vi "Update Unicode Controls.vi"(8 "error in":errorcluster, 11 "String Refs":refnum<vi>[](array[refnum])) -> (0 "error out":errorcluster, 2 "Stop Event":refnum<user-event>, 3 "Value Change Event":refnum<user-event>)   [LabVIEW 2020, in "G-Unicode.lvlib"]
doc: "Launches a background task to monitor and update string controls in <b>String Refs</b> with the correct unicode value when a user types text. The caller MUST generate a user event using <b>Stop Event</b> to terminate the background task.\n\nDynamically register for <b>Value Change Event</b> to receive an event from any of the controls in <b>String Refs</b> after the unicode text has been applied. Use Read Control.vim with the ref from Value Change Event data to read the unicode text.\n\nAll controls in <b>String Refs</b> will have their Update While Typing? and Force Unicode Text properties set True."
uses:
  G-Unicode.lvlib
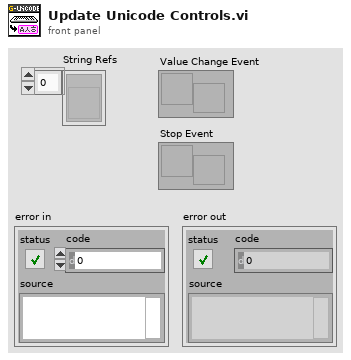
[diagram p1: front panel]
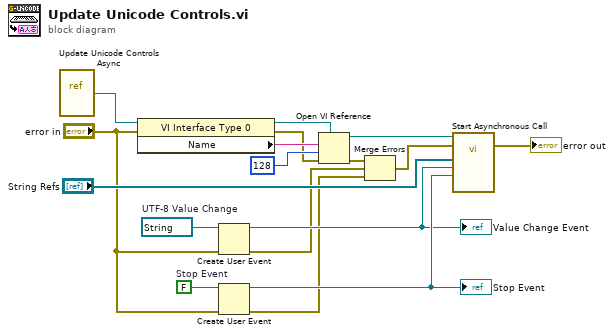
[diagram p0: block diagram]
diagram:
  w9 = refnum<vi> refnum  # UTF-8 Value Change
  w11 = FALSE  # Stop Event
  n1 = vi-ref "Update Unicode Controls Async.vi"() -> (w17:refnum<vi>)
  n2 = property class="VI Interface Type 0"(reference=w17, error in="error in") -> (reference out=w16:refnum<vi>, error out=w3:errorcluster, "Name"=w15:string)
  n3 = Create User Event(user event datatype=w9, error in="error in") -> (user event=w8:refnum<user-event>, error out=w5:errorcluster)
  "Value Change Event" <- w8
  n4 = Create User Event(user event datatype=w11, error in="error in") -> (user event=w10:refnum<user-event>, error out=w4:errorcluster)
  "Stop Event" <- w10
  n5 = Open VI Reference(type specifier VI Refnum (for type only)=w16, vi path=w15, options=128, error in (no error)=w3) -> (vi reference=w13:refnum<vi>, error out=w2:errorcluster)  [unwired: 2 in]
  n6 = Merge Errors(w2, w5, w4) -> (w1:errorcluster)
  n7 = call-by-ref "Start Asynchronous Call"(reference=w13, error in=w1, "Stop Event"=w10, "Value Change Event"=w8, "String Refs"="String Refs") -> (error out=→"error out":errorcluster)  [unwired: 9 in, 1 out]
